vi "plate control.vi"() -> ()   [LabVIEW 2015]
panel:
  in  "stop":bool
  in  "SP:":dbl(slide)=50.98039215686275 min=0.0 max=0.0 scale=0.0..100.0
  out "PV:":dbl(slide)=50.98160323470328 scale=0.0..100.0
  out "SP and PV":cluster{"initial PV":dbl, "SP1:":dbl}(graph)={"initial PV"=50.98160323470328, "SP1:"=50.98039215686275}
  in  "servo period (ms)":u32=100
  # "Proportional-Integral-Derivative (PID) Controller"
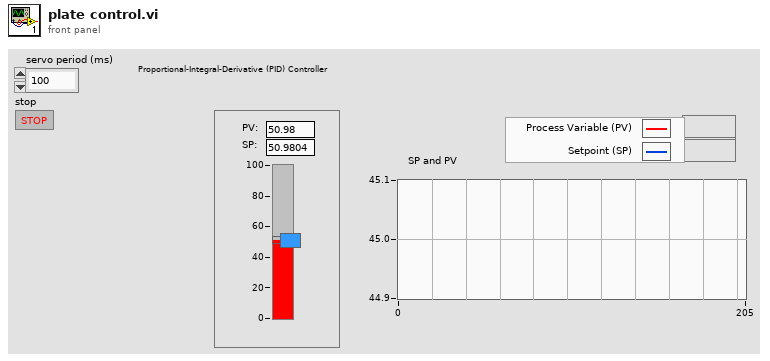
[diagram p1: front panel]
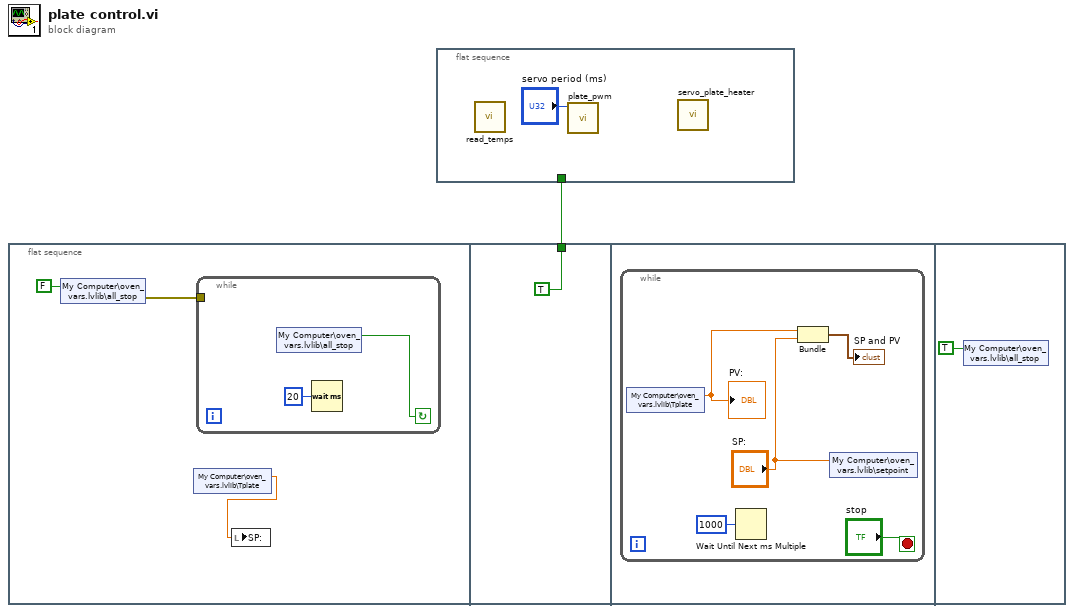
[diagram p0: block diagram]
diagram:
  n1 = flat-sequence {
    tunnel: [TRUE] -> w1
    frame #0 {
      n2 = shared-variable "My Computer\\oven_vars.lvlib\\all_stop"(FALSE ("all_stop")) -> (error out=w3:errorcluster)  [unwired: 1 in]
      n3 = shared-variable "My Computer\\oven_vars.lvlib\\Tplate"() -> (w2:dbl)  [unwired: 1 in, 1 out]
      n4 = while {
        tunnel: w3 -> [_]
        stop <- w6 continue-if-true
        n5 = shared-variable "My Computer\\oven_vars.lvlib\\all_stop"() -> (w6:bool)  [unwired: 1 in, 1 out]
        n6 = Wait (ms)(milliseconds to wait=u32 20) -> ()  [unwired: 1 out]
      }
      n7 = local write "SP:"(w2) -> ()
    }
    frame #1 {
    }
    frame #2 {
      n8 = while {
        stop <- "stop" stop-if-true
        n9 = shared-variable "My Computer\\oven_vars.lvlib\\Tplate"() -> (w11:dbl)  [unwired: 1 in, 1 out]
        "PV:" <- w11
        n10 = Wait Until Next ms Multiple(millisecond multiple=u32 1000) -> ()  [unwired: 1 out]
        n11 = Bundle("Double"=w11, "SP:"="SP:") -> (→"SP and PV":cluster{"Double":dbl, "SP:":dbl})  [unwired: 1 in]
        n12 = shared-variable "My Computer\\oven_vars.lvlib\\setpoint"("SP:") -> ()  [unwired: 1 in, 1 out]
      }
    }
    frame #3 {
      n13 = shared-variable "My Computer\\oven_vars.lvlib\\all_stop"(TRUE ("all_stop")) -> ()  [unwired: 1 in, 1 out]
    }
  }
  n14 = flat-sequence {
    tunnel: w1 -> [_]
    frame #0 {
      n15 = call "read_temps.vi"() -> ()  [unwired: 12 in]
      n16 = call "plate_pwm.vi"("period (ms)"="servo period (ms)") -> ()  [unwired: 11 in]
      n17 = call "servo_plate_heater.vi"() -> ()  [unwired: 12 in]
    }
  }
